vi "Standard Event Register Query.vi"(0 "VISA resource name":refnum<visa-resource-name>="COM1", 11 "error in (no error)":errorcluster) -> (4 "VISA resource name out":refnum<visa-resource-name>="COM1", 6 "Standard Event Register":T1, 15 "error out":errorcluster)   [LabVIEW 2020, in "Associated Research 78XX Series.lvlib"]
doc: "Queries the Event Status Register and returns the byte data available in it.\nEach bit represent the occurrence of an event.\n\nEx : BIT 0 is set High when \"Operation Complete\"\n\nBIT 0 ,01H, (1) Operation Complete\nBIT 1 ,02H, (2) Not Used\nBIT 2 ,04H, (4) Query Error\nBIT 3 ,08H, (8) Device Error\nBIT 4 ,10H,(16) Execution Error\nBIT 5 ,20H,(32) Command Error\nBIT 6 ,40H,(64) Not Used\nBIT 7 ,80H,(128) Power On"
uses:
  <instrlib>/Associated Research 78XX Series/Associated Research 78XX Series.lvlib
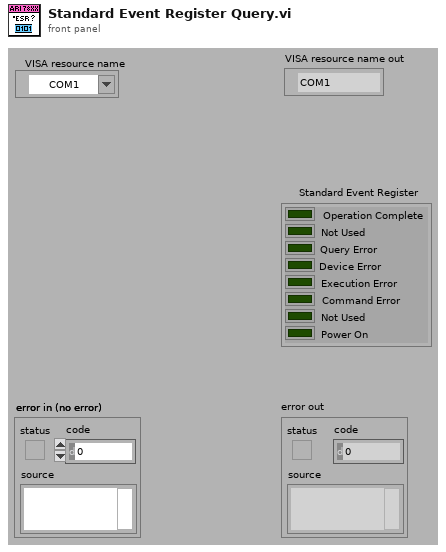
[diagram p1: front panel]
types:
  T1 = cluster{"Operation Complete":bool, "Not Used":bool, "Query Error":bool, "Device Error":bool, "Execution Error":bool, "Command Error":bool, "Not Used":bool, "Power On":bool}
  T2 = cluster{"Boolean array[0]":bool, "Boolean array[1]":bool, "Boolean array[2]":bool, "Boolean array[3]":bool, "Boolean array[4]":bool, "Boolean array[5]":bool, "Boolean array[6]":bool, "Boolean array[7]":bool}
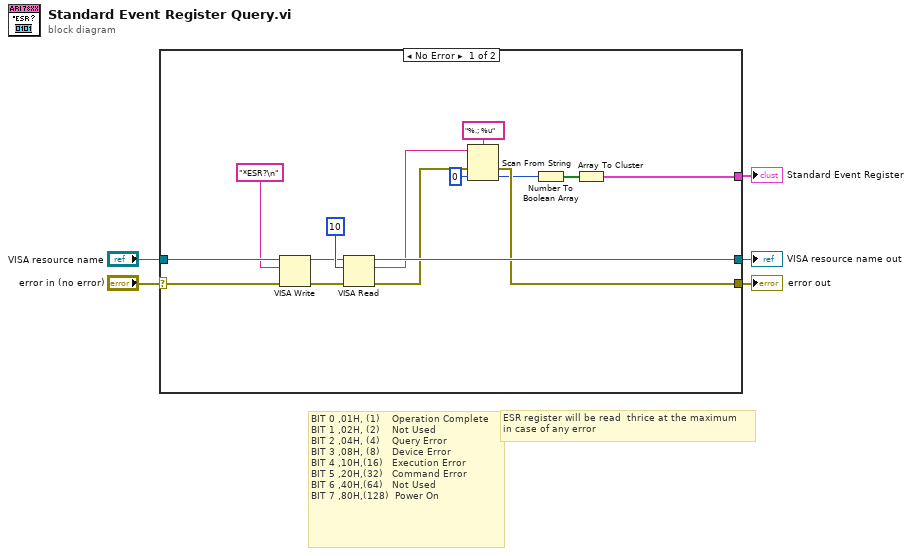
[diagram p0: block diagram]
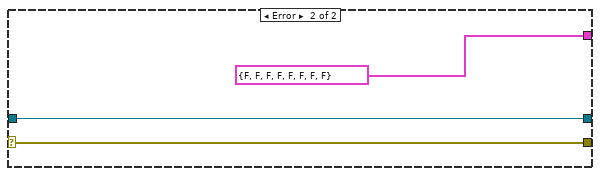
[diagram p2: hidden frame]
diagram:
  # "ESR register will be read  thrice at the maximum\nin case of any error"
  # "BIT 0 ,01H, (1)    Operation Complete\nBIT 1 ,02H, (2)    Not Used\nBIT 2 ,04H, (4)    Query Error\nBIT 3 ,08H, (8)    Device Error\nBIT 4 ,10H,(16)   Execution Error\nBIT 5 ,20H,(32)   Command Error\nBIT 6 ,40H,(64)   Not Used\nBIT 7 ,80H,(128)  Power On"
  n1 = case shown="No Error" "error in (no error)" {
    selector: "error in (no error)" -> [w17 w23]
    tunnel: [w20 T2 {"Boolean array[0]"=FALSE, "Boolean array[1]"=FALSE, "Boolean array[2]"=FALSE, "Boolean array[3]"=FALSE, "Boolean array[4]"=FALSE, "Boolean array[5]"=FALSE, "Boolean array[6]"=FALSE, "Boolean array[7]"=FALSE} ("Boolean array")] -> w1
    tunnel: [w18 w23] -> w2
    tunnel: "VISA resource name" -> [w16 w22]
    tunnel: [w19 w22] -> w4
    frame No Error {
      n2 = VISA Write(VISA resource name=w16, write buffer="*ESR?\n" ("Command to Send (empty)"), error in (no error)=w17) -> (VISA resource name out=w6:refnum<visa-resource-name>, error out=w7:errorcluster)  [unwired: 1 out]
      n3 = VISA Read(VISA resource name=w6, byte count=u32 10, error in (no error)=w7) -> (VISA resource name out=w19:refnum<visa-resource-name>, read buffer=w13:string, error out=w9:errorcluster)  [unwired: 1 out]
      n4 = Scan From String(format string="%.; %u" ("Format String"), input string=w13, error in=w9, default 1=u8 0 ("default value 1")) -> (error out=w18:errorcluster, output 1=w10:u8)  [unwired: 1 in, 2 out]
      n5 = Number To Boolean Array(number=w10) -> (Boolean array=w12:bool[])
      n6 = Array To Cluster(array=w12) -> (cluster=w20:T2)
    }
    frame Error {
    }
  }
  "Standard Event Register" <- w1
  "VISA resource name out" <- w4
  "error out" <- w2
